vi "Server Example1.vi"() -> ()   [LabVIEW 2021]
doc: "Demonstrates how to use Modbus functions to create a slave listening to a specific TCP port. It shows an interactive UI to allow users read and write the coils on a virtual slave device. Users can also get the count of masters connected to this slave."
uses:
  Sockets/VISA TCP Socket/VISA TCP.lvclass/VISA TCP.ctl
  WebSockets/WebSocket/WebSocket.lvclass/WebSocket.ctl
  WebSockets/WebSocket Server/TCP Server/TCP Server.lvclass/TCP Server.ctl
  Sockets/VISA TCP Socket/Write port.vi
  Sockets/VISA TCP Socket/Write connect timeout.vi
  WebSockets/WebSocket/Write read operation timeout.vi
  WebSockets/WebSocket/Write write operation timeout.vi
  WebSockets/WebSocket Server/TCP Server/TCP Server.lvclass
  Sockets/VISA TCP Socket/VISA TCP.lvclass
  WebSockets/Data Model/WebSocket Data Model.lvclass
  WebSockets/WebSocket/WebSocket.lvclass
  <vilib>/addons/Tools/Unicode/UTF8 Tools.lvlib
  D:/my_projects/projects/Algorithms/Labview/21/WebSockets/Sockets/Socket/Socket.lvclass
  D:/my_projects/projects/Algorithms/Labview/21/WebSockets/Sockets/VISA TCP Socket/VISA TCP.lvclass
  D:/my_projects/projects/Algorithms/Labview/21/WebSockets/WebSockets/WebSocket Server/WebSocket Server.lvclass
  D:/my_projects/projects/Algorithms/Labview/21/WebSockets/WebSockets/WebSocket/WebSocket.lvclass
  D:/my_projects/projects/Algorithms/Labview/21/WebSockets/WebSockets/WebSocket Server/TCP Server/TCP Server.lvclass
  D:/my_projects/projects/Algorithms/Labview/21/Modbus_v121c/Data Model/Device Data Model.lvclass
  D:/my_projects/projects/Algorithms/Labview/21/WebSockets/WebSockets/Data Model/WebSocket Data Model.lvclass
panel:
  out "Chart":dbl(graph)
  out "read data":string
  in  "Port":u16=6123
  in  "write period":u32=20
  out "timer":u32(graph)
  in  "Write":bool
  in  "String":string
  out "Number of Masters":u32
  in  "Stop":bool
  in  "read period":i32=20
  # "Overview: Demonstrates the use of the WebSocket Server VIs to create a WebSocket Server and read and write text and binary data on this WebSocket Server.\nInstructions:\n1. Ensure Port 6123 is not in use.\n2. Run the VI.\n3. Click Stop to stop the VI."
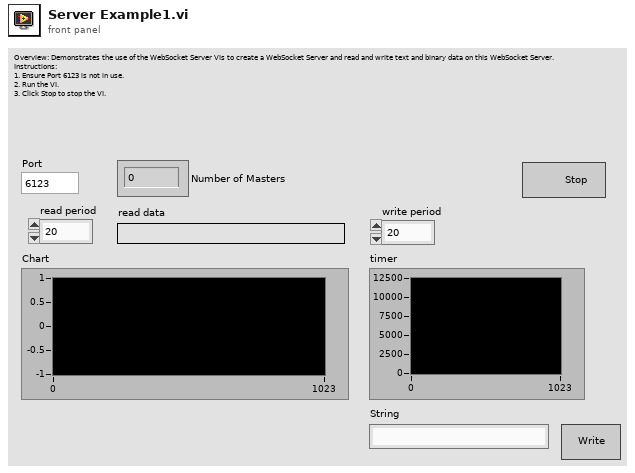
[diagram p1: front panel]
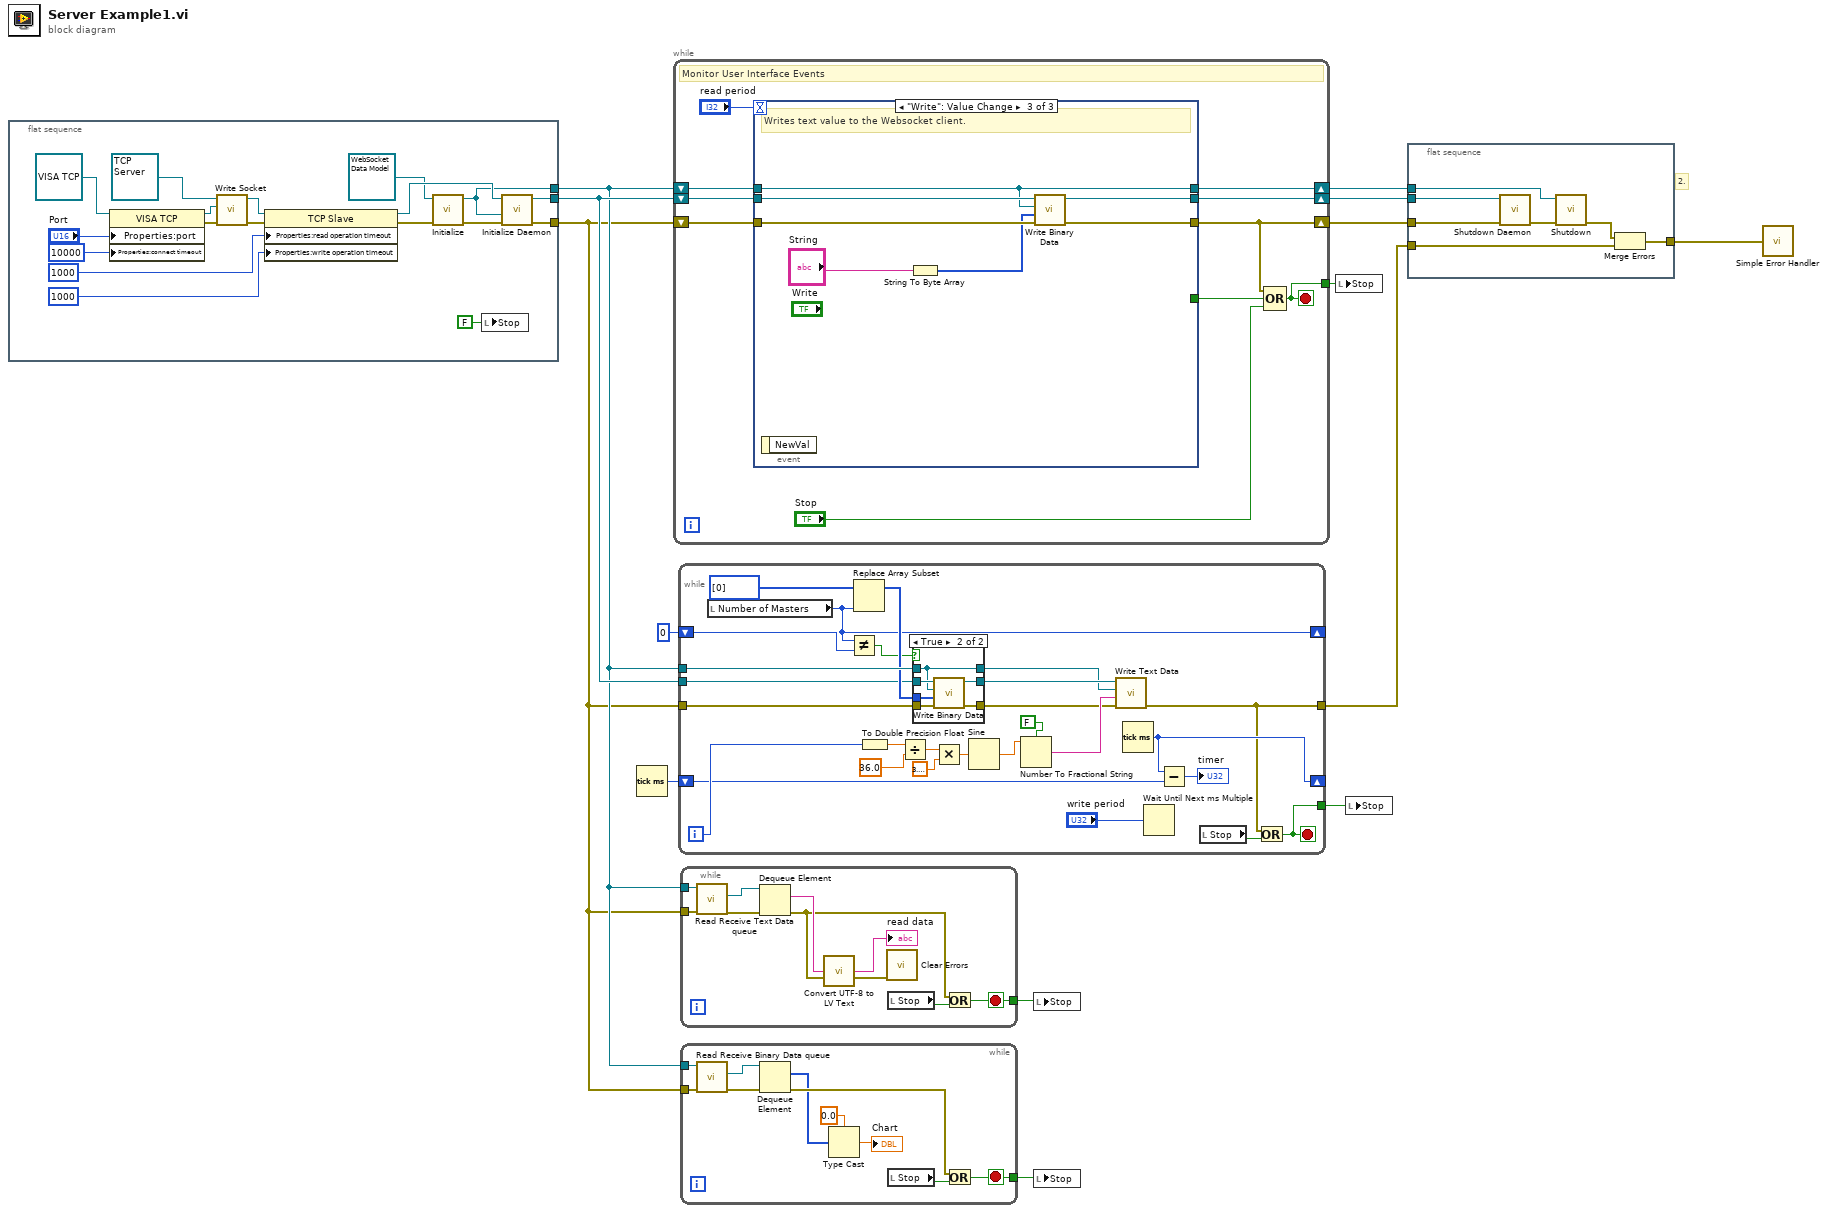
[diagram p0: block diagram]
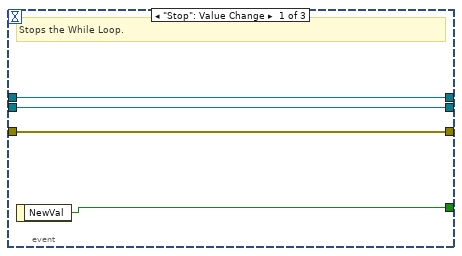
[diagram p3: hidden frame]
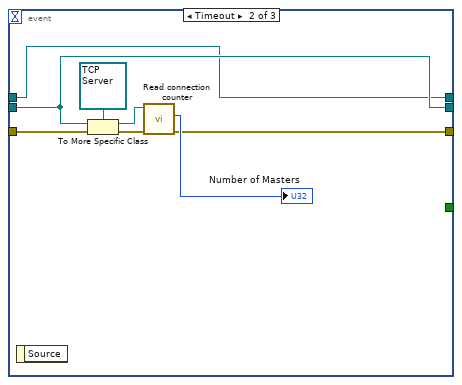
[diagram p4: hidden frame]
diagram:
  # "2."
  n1 = flat-sequence {
    tunnel: [w18] -> w1
    tunnel: [w17] -> w5
    tunnel: [w16] -> w2
    frame #0 {
      n2 = property class="VISA TCP"(reference=refnum<class "VISA TCP.lvclass"> refnum ("Sockets:VISA TCP"), "Properties:port"="Port", "Properties:connect timeout"=10000 ("connect timeout")) -> (reference out=w27:refnum<class "VISA TCP.lvclass">, error out=w28:errorcluster)  [unwired: 1 in]
      n3 = call "Write Socket.vi"("error in (no error)"=w28, "Socket"=w27, "WebSocket in"=refnum<class "TCP Server.lvclass"> refnum ("WebSockets.lvlib:TCP Slave")) -> ("error out"=w26:errorcluster, "WebSocket out"=w25:refnum<class "TCP Server.lvclass">)  [unwired: 7 in]
      n4 = property class="TCP Slave"(reference=w25, error in=w26, "Properties:read operation timeout"=1000 ("read operation timeout"), "Properties:write operation timeout"=1000 ("write operation timeout")) -> (reference out=w24:refnum<class "TCP Server.lvclass">, error out=w21:errorcluster)
      n5 = call-dynamic "Initialize.vi"("error in (no error)"=w21, "device data model in"=refnum<class "WebSocket Data Model.lvclass"> refnum ("WebSockets.lvlib:Device Data Model")) -> ("error out"=w20:errorcluster, "device data model out"=w16:refnum<class "WebSocket Data Model.lvclass">)  [unwired: 8 in]
      n6 = local write "Stop"(FALSE ("Stop")) -> ()
      n7 = call-dynamic "Initialize Daemon.vi"("error in"=w20, "Data Model"=w16, "TCP slave in"=w24) -> ("error out"=w18:errorcluster, "TCP slave out"=w17:refnum<class "TCP Server.lvclass">)  [unwired: 7 in]
    }
  }
  n8 = Tick Count (ms)() -> (millisecond timer value=w10:u32)
  n9 = while {
    shift-right: [w41] -> w12
    shift-left: w5 -> [w42]
    shift-right: [w39] -> w13
    shift-left: w1 -> [w40]
    shift-right: [w37] -> w14
    shift-left: w2 -> [w38]
    tunnel: [w33] -> w8
    stop <- w33 stop-if-true
    # "Monitor User Interface Events"
    n10 = event shown="[2] \"Write\": Value Change" {
      selector: _ -> [_ _ _]
      dyn-events: _ -> [_ _ _]
      timeout: "read period" -> [_ _ _]
      tunnel: w42 -> [w45 w50 w60]
      tunnel: [w45 w50 w59] -> w41
      tunnel: w40 -> [w46 w49 w58]
      tunnel: [w46 w48 w57] -> w39
      tunnel: w38 -> [w44 w47 w55]
      tunnel: [w44 w47 w55] -> w37
      tunnel: [w43 _ _] -> w34
      event "Stop": Value Change {
        # "Stops the While Loop."
        n11 = event-data() -> ("NewVal"=w43:bool)  [unwired: 1 in]
      }
      event Timeout {
        n12 = event-data() -> ()  [unwired: 1 in, 1 out]
        n13 = To More Specific Class(target class=refnum<class "TCP Server.lvclass"> refnum ("TCP Slave in"), reference=w50, error in=w49) -> (specific class reference=w52:refnum<class "TCP Server.lvclass">, error out=w53:errorcluster)
        n14 = call "Read connection counter.vi"("error in (no error)"=w53, "TCP Slave in"=w52) -> ("error out"=w48:errorcluster, "Currently Connected"=→"Number of Masters":u32)  [unwired: 7 in, 1 out]
      }
      event "Write": Value Change {
        # "Writes text value to the Websocket client."
        n15 = event-data() -> ()  [unwired: 1 in, 1 out]
        n16 = String To Byte Array(string="String") -> (unsigned byte array=w56:u8[])
        n17 = call-dynamic "Write Binary Data.vi"("error in (no error)"=w58, "Binary Data"=w56, "Device Data Model"=w55, "WebSocket in"=w60) -> ("error out"=w57:errorcluster, "WebSocket out"=w59:refnum<class "TCP Server.lvclass">)  [unwired: 6 in]
      }
    }
    n18 = Compound Arithmetic op=OR(w39, w34, "Stop") -> (w33:bool)
  }
  n19 = while {
    tunnel: w5 -> [w67]
    tunnel: w1 -> [w66]
    tunnel: w2 -> [w73]
    tunnel: [w62] -> w7
    tunnel: [w78] -> w11
    shift-right: [w74] -> _
    shift-left: w10 -> [w75]
    shift-right: [w70] -> _
    shift-left: u32 0 ("Number of Masters") -> [w69]
    i -> [w81]
    stop <- w78 stop-if-true
    n20 = local read "Number of Masters"() -> (w70:u32)
    n21 = Not Equal?(x=w70, y=w69) -> (x != y?=w68:bool)
    n22 = Replace Array Subset(array=u8[] [0] ("Binary Data"), new element=w70) -> (w71:u8[])  [unwired: 1 in]
    n23 = To Double Precision Float(number=w81) -> (double precision float=w88:dbl)
    n24 = Divide(x=w88, y=36.0) -> (x/y=w86:dbl)
    n25 = case shown="True" w68 {
      tunnel: w66 -> [w91 w97]
      tunnel: w73 -> [w90 w92]
      tunnel: w67 -> [w89 w96]
      tunnel: w71 -> [_ w95]
      tunnel: [w91 w94] -> w63
      tunnel: [w89 w93] -> w65
      tunnel: [w90 w92] -> w64
      frame False {
      }
      frame True {
        n26 = call-dynamic "Write Binary Data.vi"("error in (no error)"=w97, "Binary Data"=w95, "Device Data Model"=w92, "WebSocket in"=w96) -> ("error out"=w94:errorcluster, "WebSocket out"=w93:refnum<class "TCP Server.lvclass">)  [unwired: 6 in]
      }
    }
    n27 = Multiply(x=w86, y=3.141592653589793) -> (x*y=w84:dbl)
    n28 = Sine(x=w84) -> (sin(x)=w83:dbl)
    n29 = Number To Fractional String(use system decimal point (T)=FALSE, number=w83) -> (F-format string=w79:string)  [unwired: 2 in]
    n30 = call-dynamic "Write Text Data.vi"("error in (no error)"=w63, "String Data"=w79, "Device Data Model"=w64, "WebSocket in"=w65) -> ("error out"=w62:errorcluster)  [unwired: 6 in, 1 out]
    n31 = Tick Count (ms)() -> (millisecond timer value=w74:u32)
    n32 = Wait Until Next ms Multiple(millisecond multiple="write period") -> ()  [unwired: 1 out]
    n33 = Subtract(x=w74, y=w75) -> (x-y=→"timer":u32)
    n34 = local read "Stop"() -> (w80:bool)
    n35 = Or(x=w62, y=w80) -> (x .or. y?=w78:bool)
  }
  n36 = while {
    tunnel: w1 -> [w99]
    tunnel: w2 -> [w98]
    tunnel: [w106] -> w4
    stop <- w106 stop-if-true
    n37 = call "Read Receive Text Data queue.vi"("error in (no error)"=w99, "WebSocket Data Model in"=w98) -> ("error out"=w104:errorcluster, "Receive Text Data"=w105:refnum<queue>)  [unwired: 7 in, 1 out]
    n38 = Dequeue Element(queue=w105, error in (no error)=w104) -> (element=w101:string, error out=w100:errorcluster)  [unwired: 1 in, 2 out]
    n39 = call <vilib>:"Convert UTF-8 to LV Text.vi"("UTF-8 Text"=w101, "error in"=w100) -> ("LV Text"=→"read data":string, "error out"=w102:errorcluster)  [unwired: 12 in]
    n40 = call <vilib>:"Clear Errors.vi"("error in (no error)"=w102) -> ()  [unwired: 5 in, 2 out]
    n41 = local read "Stop"() -> (w107:bool)
    n42 = Or(x=w100, y=w107) -> (x .or. y?=w106:bool)
  }
  n43 = while {
    tunnel: [w116] -> w3
    tunnel: w2 -> [w112]
    tunnel: w1 -> [w111]
    stop <- w116 stop-if-true
    n44 = call "Read Receive Binary Data queue.vi"("error in (no error)"=w111, "WebSocket Data Model in"=w112) -> ("error out"=w114:errorcluster, "Receive Binary Data"=w113:refnum<queue>)  [unwired: 7 in, 1 out]
    n45 = Dequeue Element(queue=w113, error in (no error)=w114) -> (element=w108:u8[], error out=w115:errorcluster)  [unwired: 1 in, 2 out]
    n46 = Type Cast(type=0.0 ("x"), x=w108) -> (*(type *) &x=→"Chart":dbl)
    n47 = local read "Stop"() -> (w117:bool)
    n48 = Or(x=w115, y=w117) -> (x .or. y?=w116:bool)
  }
  n49 = local write "Stop"(w4) -> ()
  n50 = local write "Stop"(w3) -> ()
  n51 = local write "Stop"(w8) -> ()
  n52 = local write "Stop"(w11) -> ()
  n53 = flat-sequence {
    tunnel: w14 -> [w124]
    tunnel: w13 -> [w123]
    tunnel: w12 -> [w121]
    tunnel: w7 -> [w119]
    tunnel: [w118] -> w6
    frame #0 {
      n54 = call-dynamic "Shutdown Daemon.vi"("error in"=w123, "TCP slave in"=w121) -> ("error out"=w122:errorcluster)  [unwired: 9 in]
      n55 = call-dynamic "Shutdown.vi"("error in (no error)"=w122, "device data model in"=w124) -> ("error out"=w120:errorcluster)  [unwired: 9 in]
      n56 = Merge Errors(w120, w119) -> (w118:errorcluster)
    }
  }
  n57 = call <vilib>:"Simple Error Handler.vi"("error in (no error)"=w6) -> ()  [unwired: 4 in, 5 out]
